vi "Test Connection.vi"(8 "error in":errorcluster, 11 "Node Ptr":T1=18446744073709551615 format="%.0x") -> (0 "error out":errorcluster)   [LabVIEW 2019, in "OPC UA Client Addon System Explorer.lvlib"]
uses:
  OPC UA Client Addon System Explorer.lvlib
  <vilib>/NI VeriStand/Custom Device API/Custom Device Item Ref.ctl
  Addon Shared/SubVIs/OPCConnection.BuildURL.vi
  SubVIs/OPCConnection.Properties.vi
  <vilib>/Utility/cursorutil.llb/Set Busy.vi
  Addon Shared/SubVIs/Constants.vi
  <vilib>/NI VeriStand/Custom Device API/NI VeriStand - Get Item Property.vi
  <vilib>/NI VeriStand/Custom Device API/Get Item Property (String).vi
  <vilib>/NI VeriStand/Custom Device API/Get Item Property (U16).vi
  <vilib>/NI VeriStand/Custom Device API/Get Item Property (Dependent File).vi
  <vilib>/NI VeriStand/Custom Device API/NI VeriStand - Set Item Property.vi
  <vilib>/NI VeriStand/Custom Device API/Set Item Property (String).vi
  <vilib>/NI VeriStand/Custom Device API/Set Item Property (U16).vi
  <vilib>/Utility/libraryn.llb/Get File Extension.vi
  <vilib>/Utility/MD5Checksum.llb/MD5Checksum File.vi
  <vilib>/NI VeriStand/Custom Device API/Set Item Property (Dependent File).vi
  <vilib>/Utility/libraryn.llb/Check if File or Folder Exists.vi
  <vilib>/NI VeriStand/Custom Device API/NI VeriStand - Remove Item Property.vi
  <vilib>/OPCUA/client/Connect.vi
  <vilib>/OPCUA/client/Disconnect.vi
  <vilib>/Utility/error.llb/Simple Error Handler.vi
  <vilib>/Utility/cursorutil.llb/Unset Busy.vi
  <vilib>/NI VeriStand/Custom Device API/Custom Device API.lvlib
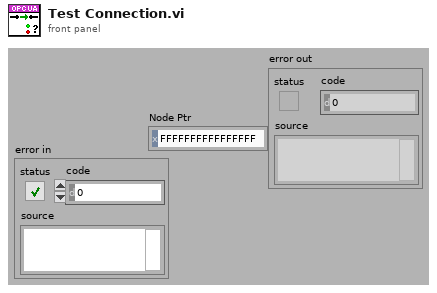
[diagram p1: front panel]
types:
  T1 = typedef "Custom Device API.lvlib/Custom Device Item Ref.ctl" = u64
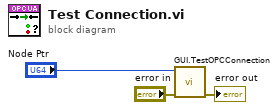
[diagram p0: block diagram]
diagram:
  n1 = call "GUI.TestOPCConnection.vi"("error in"="error in", "Node Ptr"="Node Ptr") -> ("error out"=→"error out":errorcluster)  [unwired: 9 in]
